vi "PM103 Scope Sample HW Trigger.vi"() -> ()   [LabVIEW 2019]
panel:
  out "TriggerForced":bool
  out "Scope":cluster{"Time Stamps":sgl[], "Values":sgl[]}(graph)
  in  "Autoset":bool
  out "Active":bool
  in  "stop":bool
  # "Thorlabs Power Meter Series\n       PM103 Scope HW Trigger"
  # "This example will connect the first found power meter.\nIn this example is important that the power meter has the right power range and trigger level for the light source. Press 'AUTOSET' to set the right settings.\nTo use this sample you need a PM103 with a photodiode sensor."
  # "Connected"
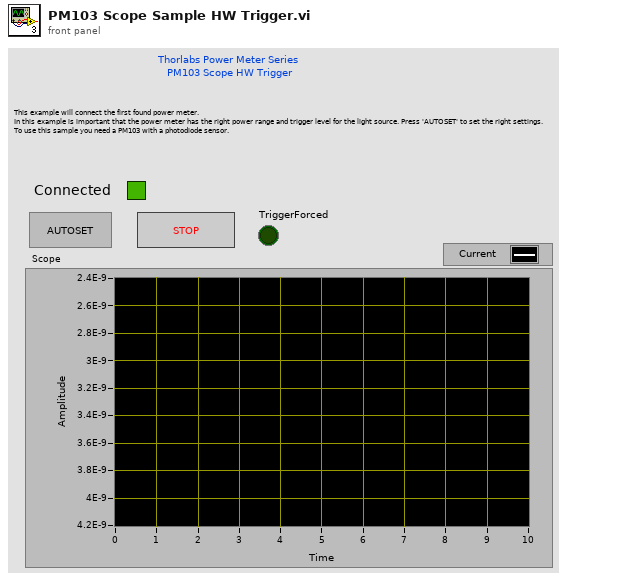
[diagram p1: front panel]
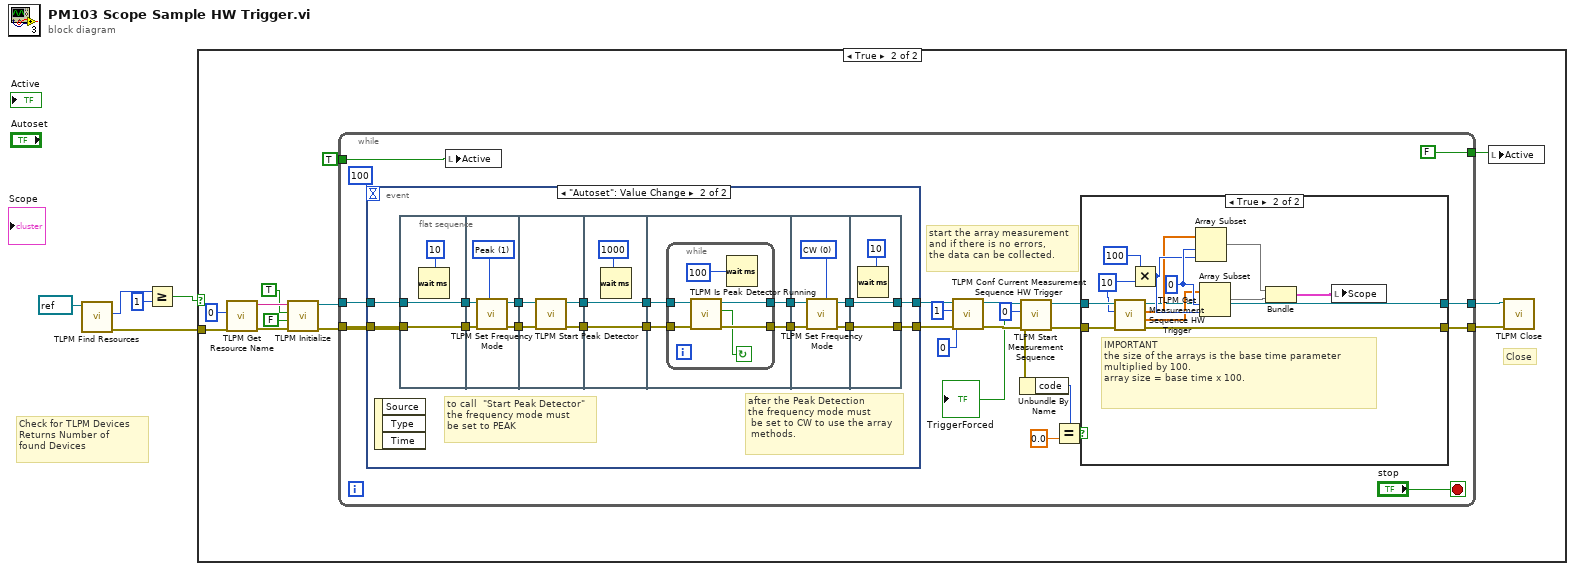
[diagram p0: block diagram]
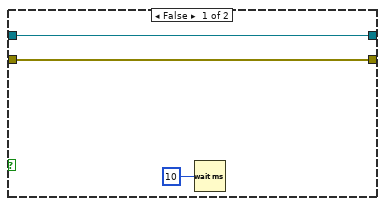
[diagram p3: hidden frame]
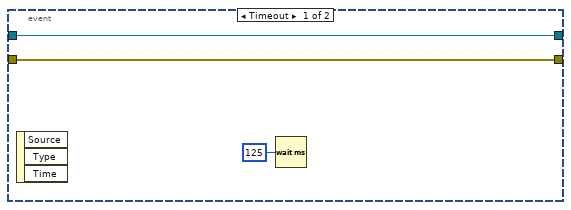
[diagram p4: hidden frame]
diagram:
  # "Check for TLPM Devices\nReturns Number of\nfound Devices"
  n1 = call <instrlib>:"TLPM Find Resources.vi"("instrument handle"=refnum<visa-resource-name> refnum) -> ("error out"=w1:errorcluster, "Resource Count"=w2:u32)  [unwired: 8 in, 1 out]
  n2 = Greater Or Equal?(x=w2, y=u32 1) -> (x >= y?=w3:bool)
  n3 = case shown="True" w3 {
    tunnel: w1 -> [_ w17]
    frame False {
    }
    frame True {
      # "Close"
      n4 = call <instrlib>:"TLPM Get Resource Name.vi"("error in (no error)"=w17, "Index (0)"=u32 0) -> ("error out"=w12:errorcluster, "Resource Name"=w15:string)  [unwired: 7 in, 1 out]
      n5 = call <instrlib>:"TLPM Initialize.vi"("error in (no error)"=w12, "Reset Device (Reset Device)"=FALSE, "ID Query (Do Query)"=TRUE, "resource name"=w15) -> ("error out"=w6:errorcluster, "instrument handle out"=w7:refnum<visa-resource-name>)  [unwired: 6 in]
      n6 = while {
        tunnel: w7 -> [w37]
        tunnel: w6 -> [w36]
        tunnel: [w30] -> w11
        tunnel: [w29] -> w10
        tunnel: TRUE -> [w28]
        tunnel: [FALSE] -> w8
        stop <- "stop" stop-if-true
        # "start the array measurement\nand if there is no errors,\nthe data can be collected."
        n7 = event shown="[1] \"Autoset\": Value Change" {
          selector: _ -> [_ _]
          dyn-events: _ -> [_ _]
          timeout: 100 -> [_ _]
          tunnel: w37 -> [w57 w73]
          tunnel: w36 -> [w56 w72]
          tunnel: [w57 w69] -> w24
          tunnel: [w56 w68] -> w23
          event Timeout {
            n8 = event-data() -> ()  [unwired: 1 in, 3 out]
            n9 = Wait (ms)(milliseconds to wait=u32 125) -> ()  [unwired: 1 out]
          }
          event "Autoset": Value Change {
            # "after the Peak Detection \nthe frequency mode must\n be set to CW to use the array\n methods."
            # "to call  \"Start Peak Detector\"\nthe frequency mode must \nbe set to PEAK"
            n10 = event-data() -> ()  [unwired: 1 in, 3 out]
            n11 = flat-sequence {
              tunnel: w73 -> [w75]
              tunnel: w72 -> [w76]
              tunnel: [w75] -> w63
              tunnel: [w76] -> w61
              tunnel: w63 -> [w77]
              tunnel: [w78] -> w62
              tunnel: w61 -> [w80]
              tunnel: [w79] -> w60
              tunnel: w62 -> [w85]
              tunnel: w60 -> [w84]
              tunnel: [w83] -> w67
              tunnel: [w82] -> w65
              tunnel: w67 -> [w88]
              tunnel: [w88] -> w66
              tunnel: w65 -> [w87]
              tunnel: [w87] -> w64
              tunnel: w66 -> [w91]
              tunnel: w64 -> [w92]
              tunnel: [w90] -> w71
              tunnel: [w89] -> w70
              tunnel: w71 -> [w102]
              tunnel: w70 -> [w101]
              tunnel: [w100] -> w59
              tunnel: [w99] -> w58
              tunnel: [w105] -> w69
              tunnel: [w106] -> w68
              tunnel: w59 -> [w106]
              tunnel: w58 -> [w105]
              frame #0 {
                n12 = Wait (ms)(milliseconds to wait=u32 10) -> ()  [unwired: 1 out]
              }
              frame #1 {
                w81 = u16 1 items=["CW", "Peak"] ("Frequency Mode (Peak)")
                n13 = call <instrlib>:"TLPM Set Frequency Mode.vi"("error in (no error)"=w80, "Frequency Mode (Peak)"=w81, "instrument handle"=w77) -> ("error out"=w79:errorcluster, "instrument handle out"=w78:refnum<visa-resource-name>)  [unwired: 7 in]
              }
              frame #2 {
                n14 = call <instrlib>:"TLPM Start Peak Detector.vi"("error in (no error)"=w84, "instrument handle"=w85) -> ("error out"=w83:errorcluster, "instrument handle out"=w82:refnum<visa-resource-name>)  [unwired: 8 in]
              }
              frame #3 {
                n15 = Wait (ms)(milliseconds to wait=u32 1000) -> ()  [unwired: 1 out]
              }
              frame #4 {
                n16 = while {
                  tunnel: w92 -> [w97]
                  tunnel: w91 -> [w96]
                  tunnel: [w95] -> w89
                  tunnel: [w94] -> w90
                  stop <- w93 continue-if-true
                  n17 = call <instrlib>:"TLPM Is Peak Detector Running.vi"("error in (no error)"=w96, "instrument handle"=w97) -> ("error out"=w95:errorcluster, "Is Running"=w93:bool, "instrument handle out"=w94:refnum<visa-resource-name>)  [unwired: 7 in]
                  n18 = Wait (ms)(milliseconds to wait=u32 100) -> ()  [unwired: 1 out]
                }
              }
              frame #5 {
                w103 = u16 0 items=["CW", "Peak"] ("Frequency Mode (Peak)")
                n19 = call <instrlib>:"TLPM Set Frequency Mode.vi"("error in (no error)"=w101, "Frequency Mode (Peak)"=w103, "instrument handle"=w102) -> ("error out"=w100:errorcluster, "instrument handle out"=w99:refnum<visa-resource-name>)  [unwired: 7 in]
              }
              frame #6 {
                n20 = Wait (ms)(milliseconds to wait=u32 10) -> ()  [unwired: 1 out]
              }
            }
          }
        }
        n21 = local write "Active"(w28) -> ()
        n22 = call <instrlib>:"TLPM Conf Current Measurement Sequence HW Trigger.vi"("error in (no error)"=w23, "Trigger Horizontal Position"=u32 0, "Averaging Limit"=u32 1, "instrument handle"=w24) -> ("error out"=w22:errorcluster, "instrument handle out"=w25:refnum<visa-resource-name>)  [unwired: 6 in]
        n23 = call <instrlib>:"TLPM Start Measurement Sequence.vi"("error in (no error)"=w22, "AutoTriggerDelay (0)"=u32 0, "instrument handle"=w25) -> ("error out"=w32:errorcluster, "TriggerForced"=→"TriggerForced":bool, "instrument handle out"=w35:refnum<visa-resource-name>)  [unwired: 6 in]
        n24 = Unbundle By Name(w32) -> ("code"=w31:i32)
        n25 = Equal?(x=w31, y=0.0) -> (x = y?=w34:bool)
        n26 = case shown="True" w34 {
          tunnel: w32 -> [w40 w53]
          tunnel: w35 -> [w41 w54]
          tunnel: [w40 w52] -> w29
          tunnel: [w41 w42] -> w30
          frame False {
            n27 = Wait (ms)(milliseconds to wait=u32 10) -> ()  [unwired: 1 out]
          }
          frame True {
            w49 = 0 ("index")
            w51 = u32 10 ("Base Time")
            # "IMPORTANT\nthe size of the arrays is the base time parameter\nmultiplied by 100.\narray size = base time x 100."
            n28 = call <instrlib>:"TLPM Get Measurement Sequence HW Trigger.vi"("error in (no error)"=w53, "Base Time"=w51, "instrument handle"=w54) -> ("error out"=w52:errorcluster, "Values"=w46:sgl[], "Time Stamps"=w47:sgl[], "instrument handle out"=w42:refnum<visa-resource-name>)  [unwired: 5 in]
            n29 = Multiply(x=u32 100, y=w51) -> (x*y=w48:u32)
            n30 = Array Subset(array=w47, index=w49, length=w48) -> (w45:sgl[])
            n31 = Array Subset(array=w46, index=w49, length=w48) -> (w44:sgl[])
            n32 = Bundle(w45, w44) -> (w43:cluster{sgl[], sgl[]})  [unwired: 1 in]
            n33 = local write "Scope"(w43) -> ()
          }
        }
      }
      n34 = local write "Active"(w8) -> ()
      n35 = call <instrlib>:"TLPM Close.vi"("error in (no error)"=w10, "instrument handle"=w11) -> ()  [unwired: 9 in, 1 out]
    }
  }
